vi "refresh scans per acquisition.vi"(8 "error in (no error)":errorcluster, 11 "LineCCD in":refnum<class "LineCCD.lvclass">) -> (0 "error out":errorcluster, 3 "LineCCD out":refnum<class "LineCCD.lvclass">)   [LabVIEW 2012, in "LineCCD.lvclass"]
uses:
  LineCCD.lvclass
  LineCCD.lvclass/LineCCD.ctl
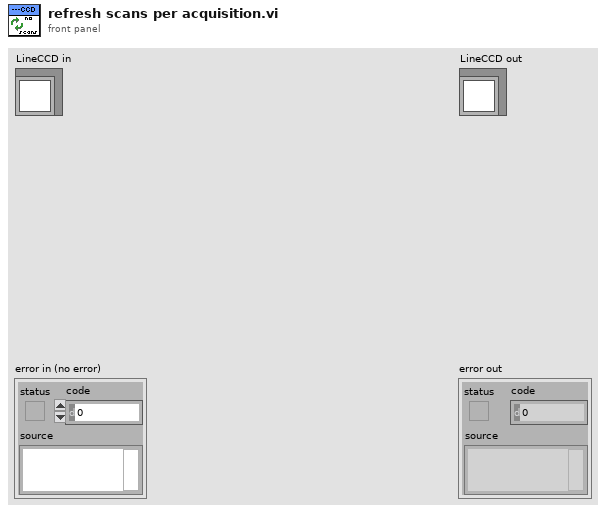
[diagram p1: front panel]
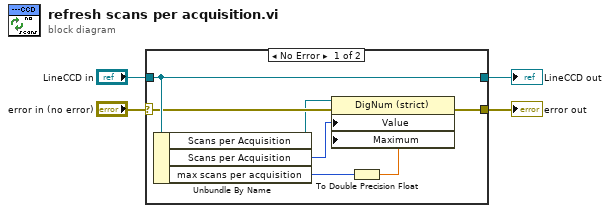
[diagram p0: block diagram]
diagram:
  n1 = case shown="No Error" "error in (no error)" {
    selector: "error in (no error)" -> [w10 w13]
    tunnel: [w9 w13] -> w3
    tunnel: [w11 w12] -> w1
    tunnel: "LineCCD in" -> [w11 w12]
    frame No Error {
      n2 = Unbundle By Name(w11) -> ("Scans per Acquisition"=w8:refnum<vi>, "Scans per Acquisition"=w7:u32, "max scans per acquisition"=w6:u32)
      n3 = To Double Precision Float(number=w6) -> (double precision float=w5:dbl)
      n4 = property class="DigNum (strict)"(reference=w8, error in=w10, "Value"=w7, "Maximum"=w5) -> (error out=w9:errorcluster)  [unwired: 1 out]
    }
    frame Error {
    }
  }
  "error out" <- w3
  "LineCCD out" <- w1
